vi "Run Selected Measurement Service.vi"(8 "error in":errorcluster, 10 "Measurement Service Names":string[](array[string]), 11 "Project ref":refnum<vi>) -> (0 "error out":errorcluster, 3 "Measurement Service Successfully run":string[](array[string]))   [LabVIEW 2020, in "MeasurementService Editor.lvlib"]
uses:
  MeasurementService Editor.lvlib
  0b32f8da-aca2-4937-8be8-c570bca556b7.vi
  <vilib>/Comparison/Equal/Equal Functor/Equal Functor.lvclass
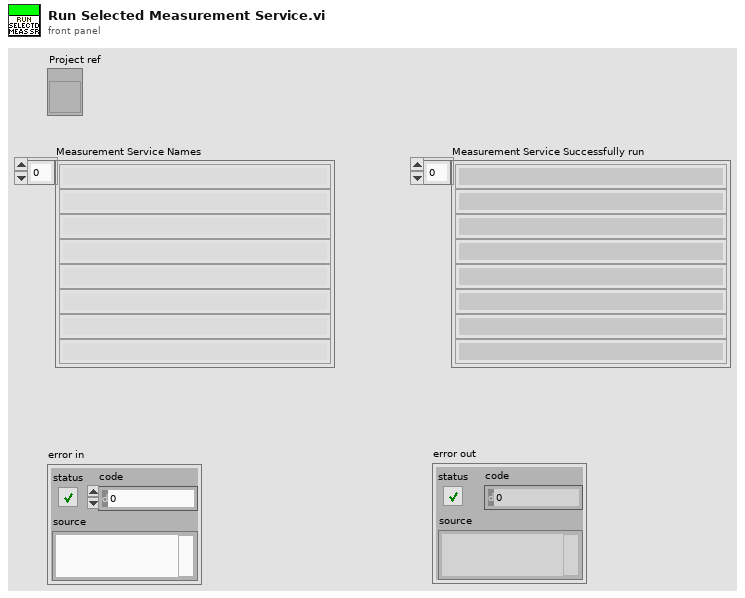
[diagram p1: front panel]
types:
  T1 = enum32{"Invalid", "Standard", "Closed", "Hidden", "Minimized", "Maximized"}
  T2 = enum32{"Bad", "Idle", "Run top level", "Running"}
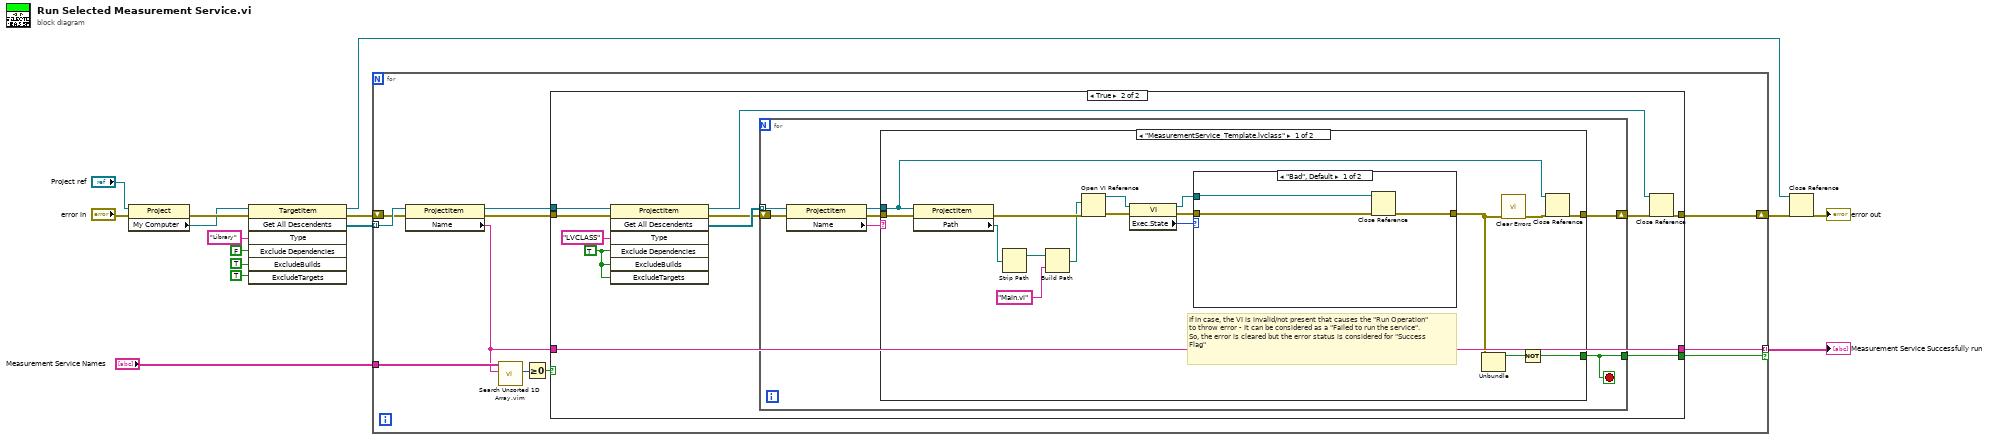
[diagram p0: block diagram]
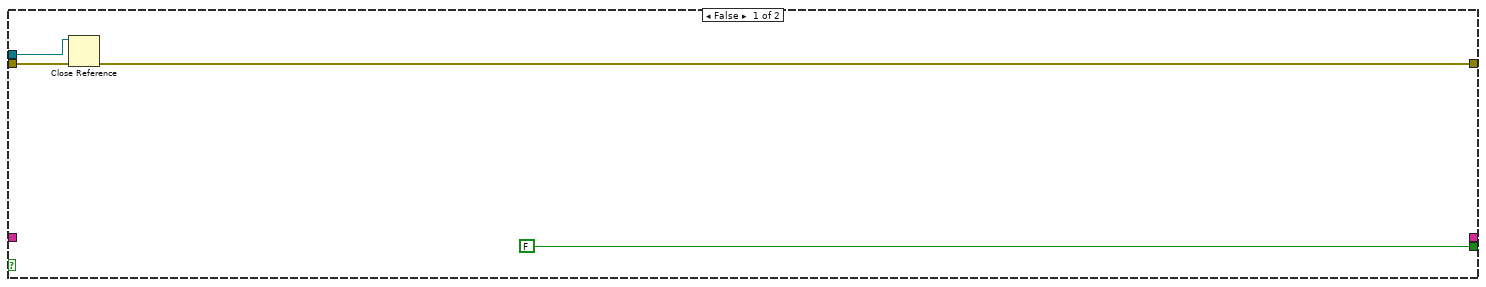
[diagram p2: hidden frame]
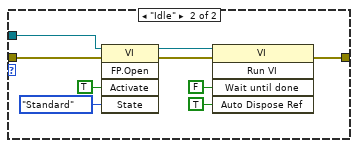
[diagram p3: hidden frame]
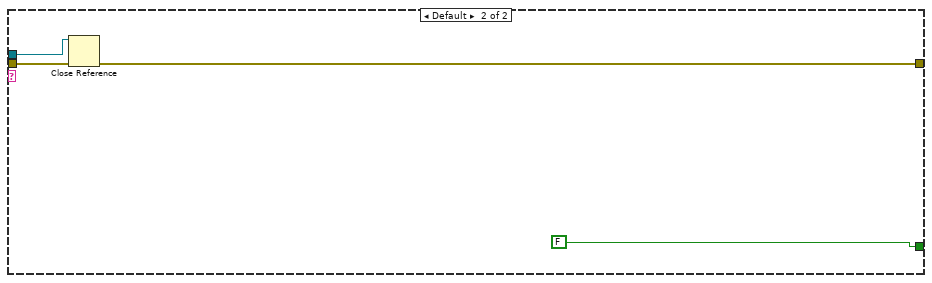
[diagram p4: hidden frame]
diagram:
  n1 = property class="Project"(reference="Project ref", error in="error in") -> (error out=w9:errorcluster, "My Computer"=w8:refnum<vi>)  [unwired: 1 out]
  n2 = invoke class="TargetItem" method="Get All Descendents"(reference=w8, error in=w9, "Type"="Library", "Exclude Dependencies"=FALSE ("ExcludeDependencies"), "ExcludeBuilds"=TRUE, "ExcludeTargets"=TRUE) -> (reference out=w4:refnum<vi>, error out=w11:errorcluster, "All Descendents"=w12:refnum<vi>[])  [unwired: 1 in, 4 out]
  n3 = for {
    tunnel: w12 -> [w26] mode=indexing
    shift-right: [w24] -> w5
    shift-left: w11 -> [w25]
    tunnel: "Measurement Service Names" -> [w21]
    tunnel: [w17] -> w1 mode=indexing if=w16
    n4 = property class="ProjectItem"(reference=w26, error in=w25) -> (reference out=w23:refnum<vi>, error out=w22:errorcluster, "Name"=w18:string)
    n5 = call "Search Unsorted 1D Array.vim"("element"=w18, "unsorted 1D array"=w21) -> ("index of element"=w20:i32)  [unwired: 9 in]
    n6 = Greater Or Equal To 0?(x=w20) -> (x >= 0?=w19:bool)
    n7 = case shown="True" w19 {
      tunnel: [w28 w41] -> w24
      tunnel: w23 -> [w29 w40]
      tunnel: w22 -> [w30 w39]
      tunnel: w18 -> [_ w32]
      tunnel: [_ w32] -> w17
      tunnel: [FALSE w31] -> w16
      frame False {
        n8 = Close Reference(reference=w29, error in (no error)=w30) -> (error out=w28:errorcluster)
      }
      frame True {
        w37 = TRUE ("ExcludeDependencies")
        n9 = invoke class="ProjectItem" method="Get All Descendents"(reference=w40, error in=w39, "Type"="LVCLASS", "Exclude Dependencies"=w37, "ExcludeBuilds"=w37, "ExcludeTargets"=w37) -> (reference out=w38:refnum<vi>, error out=w33:errorcluster, "All Descendents"=w35:refnum<vi>[])  [unwired: 1 in, 4 out]
        n10 = for {
          tunnel: w35 -> [w48] mode=indexing
          shift-right: [w45] -> w34
          shift-left: w33 -> [w44]
          tunnel: [w42] -> w31
          stop <- w42 stop-if-true
          n11 = property class="ProjectItem"(reference=w48, error in=w44) -> (reference out=w47:refnum<vi>, error out=w46:errorcluster, "Name"=w43:string)
          n12 = case shown="\"MeasurementService_Template.lvclass\"" w43 {
            tunnel: w47 -> [w63 w81]
            tunnel: w46 -> [w64 w80]
            tunnel: [w65 w79] -> w45
            tunnel: [w56 FALSE] -> w42
            frame "MeasurementService_Template.lvclass" {
              # "If in case, the VI is invalid/not present that causes the \"Run Operation\" to throw error - It can be considered as a \"Failed to run the service\". So, the error is cleared but the error status is considered for \"Success Flag\""
              n13 = property class="ProjectItem"(reference=w63, error in=w64) -> (error out=w59:errorcluster, "Path"=w61:path)  [unwired: 1 out]
              n14 = Strip Path(path=w61) -> (stripped path=w60:path)  [unwired: 1 out]
              n15 = Build Path(base path=w60, name or relative path="Main.vi") -> (appended path=w58:path)
              n16 = Open VI Reference(vi path=w58, error in (no error)=w59) -> (vi reference=w49:refnum<vi>, error out=w52:errorcluster)  [unwired: 4 in]
              n17 = property class="VI"(reference=w49, error in=w52) -> (reference out=w50:refnum<vi>, error out=w51:errorcluster, "Exec.State"=w53:T2)
              n18 = case shown="\"Bad\", Default" w53 {
                tunnel: w51 -> [w68 w72]
                tunnel: [w67 w75] -> w55
                tunnel: w50 -> [w66 w70]
                frame "Bad", Default {
                  n19 = Close Reference(reference=w66, error in (no error)=w68) -> (error out=w67:errorcluster)
                }
                frame "Idle" {
                  n20 = invoke class="VI" method="FP.Open"(reference=w70, error in=w72, "Activate"=TRUE ("Activate?"), "State"=T1."Standard") -> (reference out=w69:refnum<vi>, error out=w71:errorcluster)  [unwired: 1 in, 3 out]
                  n21 = invoke class="VI" method="Run VI"(reference=w69, error in=w71, "Wait until done"=FALSE ("Wait Until Done"), "Auto Dispose Ref"=TRUE ("Auto Dispose Reference")) -> (error out=w75:errorcluster)  [unwired: 1 in, 4 out]
                }
              }
              n22 = Unbundle(w55) -> ("status"=w57:bool)  [unwired: 2 out]
              n23 = call <vilib>:"Clear Errors.vi"("error in (no error)"=w55) -> ("error out"=w54:errorcluster)  [unwired: 5 in, 1 out]
              n24 = Not(x=w57) -> (.not. x?=w56:bool)
              n25 = Close Reference(reference=w63, error in (no error)=w54) -> (error out=w65:errorcluster)
            }
            frame Default {
              n26 = Close Reference(reference=w81, error in (no error)=w80) -> (error out=w79:errorcluster)
            }
          }
        }
        n27 = Close Reference(reference=w38, error in (no error)=w34) -> (error out=w41:errorcluster)
      }
    }
  }
  "Measurement Service Successfully run" <- w1
  n28 = Close Reference(reference=w4, error in (no error)=w5) -> (error out=→"error out":errorcluster)
